vi "StopClone.vi"(8 "error in (no error)":errorcluster, 9 "Wait for Module to stop?":bool, 11 "ModuleAdmin":refnum<class "ModuleAdmin.lvclass">) -> (0 "error out":errorcluster)   [LabVIEW 2014, in "DigitizerModule.lvlib"]
uses:
  DigitizerModule.lvlib
  <userlib>/NIST/ModuleAdminLib/ModuleAdmin/ModuleAdmin.lvclass
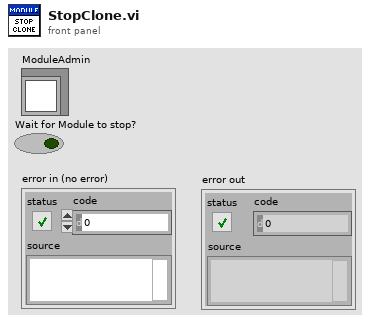
[diagram p1: front panel]
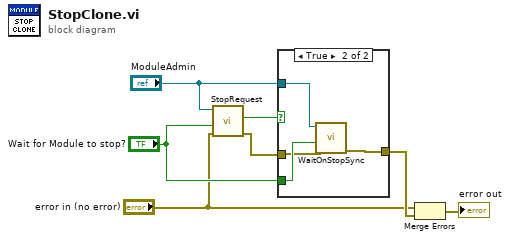
[diagram p0: block diagram]
diagram:
  n1 = call "StopRequest.vi"("error in (no error)"="error in (no error)", "Wait for Module to stop? (F)"="Wait for Module to stop?", "ModuleAdmin"="ModuleAdmin") -> ("error out"=w2:errorcluster, "Wait to Stop"=w3:bool)  [unwired: 7 in]
  n2 = case shown="True" w3 {
    tunnel: "Wait for Module to stop?" -> [_ w12]
    tunnel: [w8 w11] -> w6
    tunnel: w2 -> [w8 w10]
    tunnel: "ModuleAdmin" -> [_ w9]
    frame False {
    }
    frame True {
      n3 = call <userlib>:"WaitOnStopSync.vi"("error in (no error)"=w10, "WaitForModuleToStop?"=w12, "ModuleAdmin"=w9) -> ("error out"=w11:errorcluster)  [unwired: 7 in, 1 out]
    }
  }
  n4 = Merge Errors("error in (no error)", w6) -> (→"error out":errorcluster)
